vi "Multicast Receiver & RIO Sender.vi"() -> ()   [LabVIEW 2015]
doc: "Creates a read-only UDP multicast session and receives data on the specified port."
uses:
  <vilib>/Utility/tcp.llb/UDP Multicast Read-Only Open.vi
panel:
  out "UDP Data Value":dbl
  out "error out":errorcluster
  out "Multicast":dbl(graph)
  in  "Stop":bool
  # "Overview: Demonstrates the use of the UDP functions to connect to a UDP multicast session and receive data.\nInstructions:\n1. Ensure UDP Multicast - Sender.vi is already running.\n2. Run the VI.\n3. Click Stop to stop the VI."
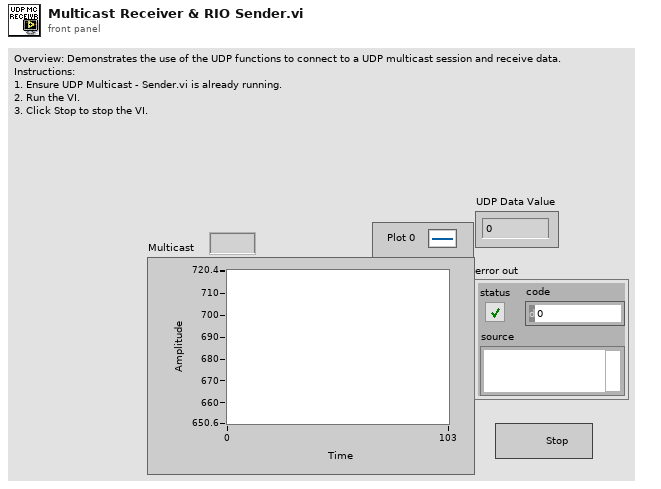
[diagram p1: front panel]
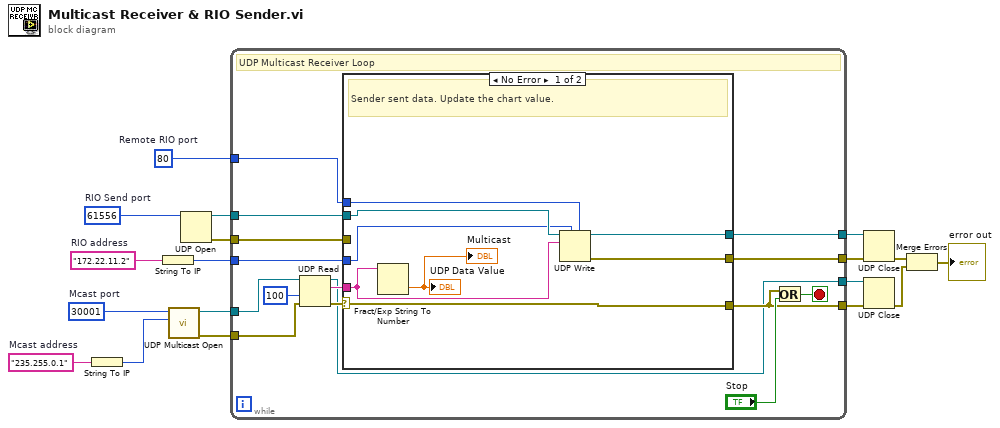
[diagram p0: block diagram]
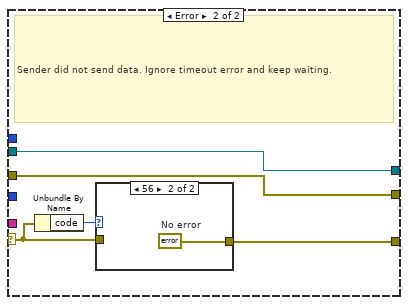
[diagram p2: hidden frame]
diagram:
  w6 = u16 80  # Remote RIO port
  w10 = u16 61556  # RIO Send port
  w11 = "172.22.11.2"  # RIO address
  w13 = u16 30001  # Mcast port
  w17 = "235.255.0.1"  # Mcast address
  n1 = String To IP(1:w17) -> (0:w12:u32)
  n2 = String To IP(1:w11) -> (0:w7:u32)
  n3 = call-poly <vilib>:"UDP Multicast Open.vi"("multicast addr"=w12, "port"=w13) -> ("error out"=w15:errorcluster, "connection ID"=w14:refnum<k16>)  [unwired: 7 in, 1 out]
  n4 = UDP Open(11:w10) -> (port=w8:refnum<k16>, 0:w9:errorcluster)  [unwired: 4 in, 1 out]
  n5 = while {
    tunnel: w14 -> [w33]
    tunnel: [w25] -> w18
    tunnel: w15 -> [w30]
    tunnel: [w26] -> w16
    tunnel: w9 -> [w19]
    tunnel: w8 -> [w24]
    tunnel: w7 -> [w23]
    tunnel: w6 -> [w22]
    tunnel: [w21] -> w5
    tunnel: [w20] -> w4
    stop <- w31 stop-if-true
    # "UDP Multicast Receiver Loop"
    n6 = UDP Read(connection ID=w33, timeout ms (25000)=100, 8:w30) -> (data out=w28:string, error out=w27:errorcluster, 3:w25:refnum<k16>)  [unwired: 3 out]
    n7 = case shown="No Error" w27 {
      selector: w27 -> [w34 w45]
      tunnel: w28 -> [w41 _]
      tunnel: [w34 w44] -> w26
      tunnel: w24 -> [w40 w43]
      tunnel: w23 -> [w39 _]
      tunnel: w22 -> [w38 _]
      tunnel: [w37 w43] -> w21
      tunnel: [w36 w42] -> w20
      tunnel: w19 -> [_ w42]
      frame No Error {
        # "Sender sent data. Update the chart value."
        n8 = Fract/Exp String To Number(string=w41) -> (number=→"Multicast" →"UDP Data Value":dbl)  [unwired: 3 in, 1 out]
        n9 = UDP Write(address=w39, port or service name=w38, connection ID=w40, data in=w41) -> (error out=w36:errorcluster, 3:w37:refnum<k16>)  [unwired: 2 in]
      }
      frame Error {
        # "Sender did not send data. Ignore timeout error and keep waiting."
        n10 = Unbundle By Name(w45) -> ("code"=w46:i32)
        n11 = case shown="56" w46 {
          tunnel: w45 -> [w47 _]
          tunnel: [w47 w48] -> w44
          frame Default {
          }
          frame 56 {
            w48 = errorcluster {"status"=FALSE, "code"=0, "source"=""}  # No error
          }
        }
      }
    }
    n12 = Or(x=w26, y="Stop") -> (x .or. y?=w31:bool)
  }
  n13 = UDP Close(connection ID=w5, 8:w4) -> (error out=w3:errorcluster)  [unwired: 1 out]
  n14 = UDP Close(connection ID=w18, 8:w16) -> (error out=w2:errorcluster)  [unwired: 1 out]
  n15 = Merge Errors(w3, w2) -> (→"error out":errorcluster)
